vi "update.vi"(8 "error in (no error)":errorcluster, 11 "ScanModeTS090821Circular2D in":refnum<class "ImagingModeTS090821Circular2D.lvclass">) -> (0 "error out":errorcluster, 3 "ScanModeTS090821Circular2D out":refnum<class "ImagingModeTS090821Circular2D.lvclass">)   [LabVIEW 2010, in "ImagingModeTS090821Circular2D.lvclass"]
uses:
  ImagingModeTS090821Circular2D.lvclass
  ImagingModeDL091001Scaffold/ImagingModeDL091001Scaffold/ImagingModeDL091001Scaffold.lvclass
  ImagingModeTS090821Circular2D.lvclass/ImagingModeTS090821Circular2D.ctl
  Trajectory/TrajectoryDL091126GenericVoxel/TrajectoryDL091126GenericVoxel/TrajectoryDL091126GenericVoxel.lvclass
  ScanHead/GenericScanHead/GenericScanHead/GenericScanHead.lvclass
  DataCollection/GenericDataCollection/GenericDataCollection/GenericDataCollection.lvclass
  ImageAssembler/GenericImageAssembler/GenericImageAssembler/GenericImageAssembler.lvclass
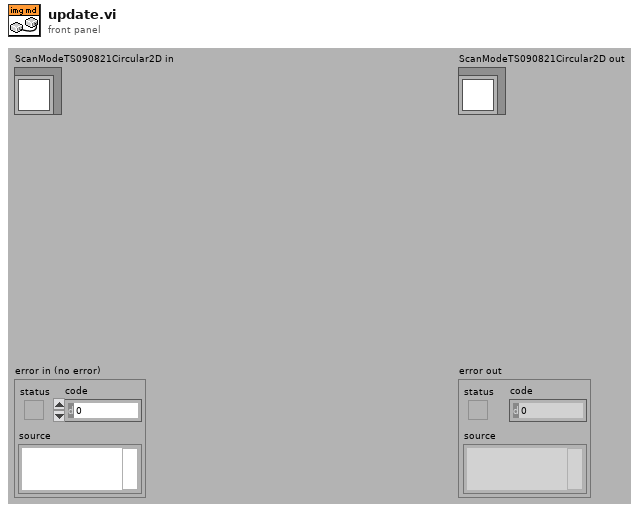
[diagram p1: front panel]
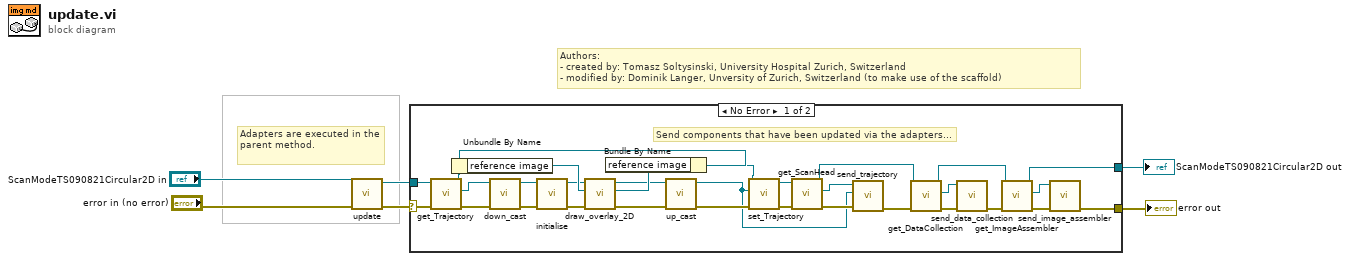
[diagram p0: block diagram]
diagram:
  # "Adapters are executed in the parent method."
  # "Authors: \n- created by: Tomasz Soltysinski, University Hospital Zurich, Switzerland\n- modified by: Dominik Langer, Unversity of Zurich, Switzerland (to make use of the scaffold)"
  n1 = call-parent "update.vi"("error in (no error)"="error in (no error)", "ScanModeDL090923Scaffold in"="ScanModeTS090821Circular2D in") -> ("error out"=w2:errorcluster, "ScanModeDL090923Scaffold out"=w1:refnum<class "ImagingModeTS090821Circular2D.lvclass">)  [unwired: 8 in]
  n2 = case shown="No Error" w2 {
    selector: w2 -> [w24 w38]
    tunnel: [w31 w38] -> w6
    tunnel: [w30 w37] -> w5
    tunnel: w1 -> [w23 w37]
    frame No Error {
      # "Send components that have been updated via the adapters..."
      n3 = call-dynamic "get_Trajectory.vi"("error in (no error)"=w24, "ScanModeDL090923Scaffold in"=w23) -> ("error out"=w16:errorcluster, "Trajectory"=w13:refnum<class "GenericTrajectory.lvclass">, "ScanModeDL090923Scaffold out"=w19:refnum<class "ImagingModeTS090821Circular2D.lvclass">)  [unwired: 2 in, 5 out]
      n4 = Unbundle By Name(w19) -> ("reference image"=w22:refnum<class "Image.lvclass">)
      n5 = call "down_cast.vi"("error in (no error)"=w16, "GenericTrajectory.lvclass"=w13) -> ("error out"=w15:errorcluster, "TrajectoryDL091126GenericVoxel out"=w12:refnum<class "TrajectoryDL091126GenericVoxel.lvclass">)  [unwired: 8 in]
      n6 = call-dynamic "initialise.vi"("error in (no error)"=w15, "GenericTrajectory in"=w12) -> ("error out"=w14:errorcluster, "GenericTrajectory out"=w11:refnum<class "TrajectoryDL091126GenericVoxel.lvclass">)  [unwired: 8 in]
      n7 = call-dynamic "draw_overlay_2D.vi"("error in (no error)"=w14, "image in"=w22, "GenericTrajectory in"=w11) -> ("error out"=w10:errorcluster, "image out"=w17:refnum<class "Image.lvclass">, "GenericTrajectory out"=w9:refnum<class "TrajectoryDL091126GenericVoxel.lvclass">)  [unwired: 6 in]
      n8 = Bundle By Name(cluster=w19, "reference image"=w17) -> (w18:refnum<class "ImagingModeTS090821Circular2D.lvclass">)
      n9 = call "up_cast.vi"("error in (no error)"=w10, "TrajectoryDL091126GenericVoxel in"=w9) -> ("error out"=w8:errorcluster, "GenericTrajectory.lvclass"=w7:refnum<class "GenericTrajectory.lvclass">)  [unwired: 8 in]
      n10 = call-dynamic "set_Trajectory.vi"("error in (no error)"=w8, "GenericTrajectory.lvclass"=w7, "ScanModeDL090923Scaffold in"=w18) -> ("error out"=w21:errorcluster, "ScanModeDL090923Scaffold out"=w20:refnum<class "ImagingModeTS090821Circular2D.lvclass">)  [unwired: 7 in]
      n11 = call-dynamic "get_ScanHead.vi"("error in (no error)"=w21, "ScanModeDL090923Scaffold in"=w20) -> ("error out"=w28:errorcluster, "ScanHead"=w27:refnum<class "GenericScanHead.lvclass">, "ScanModeDL090923Scaffold out"=w26:refnum<class "ImagingModeTS090821Circular2D.lvclass">)  [unwired: 4 in, 3 out]
      n12 = call-dynamic "send_trajectory.vi"("error in (no error)"=w28, "trajectory"=w7, "GenericScanHead in"=w27) -> ("error out"=w25:errorcluster)  [unwired: 7 in, 1 out]
      n13 = call-dynamic "get_DataCollection.vi"("error in (no error)"=w25, "ScanModeDL090923Scaffold in"=w26) -> ("error out"=w35:errorcluster, "DataCollection"=w36:refnum<class "GenericDataCollection.lvclass">, "ScanModeDL090923Scaffold out"=w29:refnum<class "ImagingModeTS090821Circular2D.lvclass">)  [unwired: 4 in, 3 out]
      n14 = call-dynamic "send_data_collection.vi"("error in (no error)"=w35, "GenericDataCollection in"=w36) -> ("error out"=w34:errorcluster)  [unwired: 8 in, 1 out]
      n15 = call-dynamic "get_ImageAssembler.vi"("error in (no error)"=w34, "ScanModeDL090923Scaffold in"=w29) -> ("error out"=w32:errorcluster, "ImageAssembler"=w33:refnum<class "GenericImageAssembler.lvclass">, "ScanModeDL090923Scaffold out"=w30:refnum<class "ImagingModeTS090821Circular2D.lvclass">)  [unwired: 4 in, 3 out]
      n16 = call-dynamic "send_image_assembler.vi"("error in (no error)"=w32, "GenericImageAssembler in"=w33) -> ("error out"=w31:errorcluster)  [unwired: 8 in, 1 out]
    }
    frame Error {
    }
  }
  "error out" <- w6
  "ScanModeTS090821Circular2D out" <- w5
